vi "Place piece.vi"(9 "Piece":refnum<class "Piece.lvclass">, 10 "Square":T1={"File"=enum."a", "Rank"=enum."4"}, 11 "Board in":refnum<class "Board.lvclass">) -> (1 "Removed piece":refnum<class "Piece.lvclass">, 2 "Square occupied?":bool, 3 "Board out":refnum<class "Board.lvclass">)   [LabVIEW 2016, in "Chesslib.lvlib" / "Board.lvclass"]
uses:
  Board.lvclass
  Pieces/Piece/Piece.lvclass
  typedef/Square.ctl
  typedef/File.ctl
  typedef/Rank.ctl
  Board.lvclass/Board.ctl
  Chesslib.lvlib
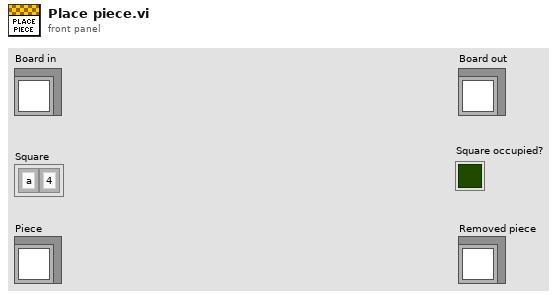
[diagram p1: front panel]
types:
  T1 = typedef "Chesslib.lvlib/Square.ctl" = cluster{"File":T2, "Rank":T3}
  T2 = typedef "Chesslib.lvlib/File.ctl" = enum8{"a", "b", "c", "d", "e", "f", "g", "h"}
  T3 = typedef "Chesslib.lvlib/Rank.ctl" = enum8{"1", "2", "3", "4", "5", "6", "7", "8"}
  T4 = typedef "Chesslib.lvlib/Board.lvclass/Square content.ctl" = cluster{"Occupied":bool, "Piece":refnum<class "Piece.lvclass">}
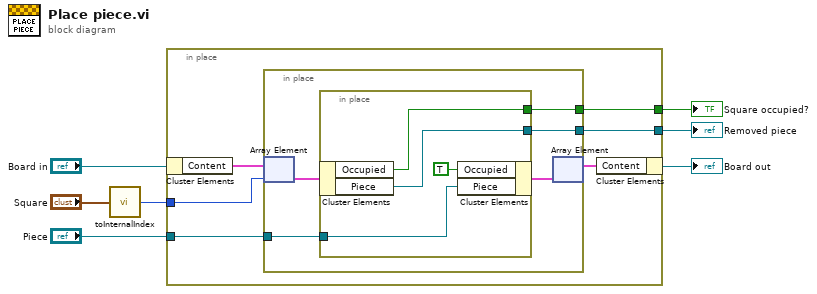
[diagram p0: block diagram]
diagram:
  n1 = call "toInternalIndex.vi"("Square"="Square") -> ("Internal index"=w5:u8)
  n2 = in-place {
    in-place-border: w5 -> [w12]
    in-place-border: "Piece" -> [w10]
    in-place-border: [w9] -> w2
    in-place-border: [w8] -> w1
    n3 = in-place-cluster #1("Board in") -> ("Content"=w13:T4[])
    n4 = in-place {
      in-place-border: w10 -> [w17]
      in-place-border: [w16] -> w9
      in-place-border: [w15] -> w8
      n5 = in-place-array #2(w13, w12) -> (w18:T4)
      n6 = in-place {
        in-place-border: w17 -> [w22]
        in-place-border: [w20] -> w16
        in-place-border: [w19] -> w15
        n7 = in-place-cluster #3(w18) -> ("Occupied"=w20:bool, "Piece"=w19:refnum<class "Piece.lvclass">)
        n8 = in-place-cluster #3("Occupied"=TRUE, "Piece"=w22) -> (w14:T4)
      }
      n9 = in-place-array #2(w14) -> (w11:T4[])  [unwired: 1 out]
    }
    n10 = in-place-cluster #1("Content"=w11) -> (→"Board out":refnum<class "Board.lvclass">)
  }
  "Square occupied?" <- w2
  "Removed piece" <- w1
